vi "Write Error Handler Actor Queue.vi"(8 "error in (no error)":errorcluster, 10 "Actor Framework.lvlib:Message Enqueuer":refnum<class "Message Enqueuer.lvclass">, 11 "Controller in":refnum<class "Controller.lvclass">) -> (0 "error out":errorcluster, 3 "Controller out":refnum<class "Controller.lvclass">)   [LabVIEW 2026, in "Controller Actor.lvlib" / "Controller.lvclass"]
uses:
  Controller.lvclass
  Controller.lvclass/Controller.ctl
  <vilib>/ActorFramework/Message Enqueuer/Message Enqueuer.lvclass
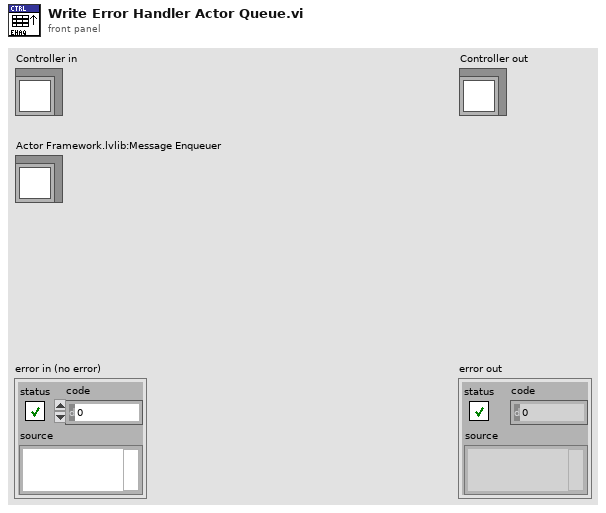
[diagram p1: front panel]
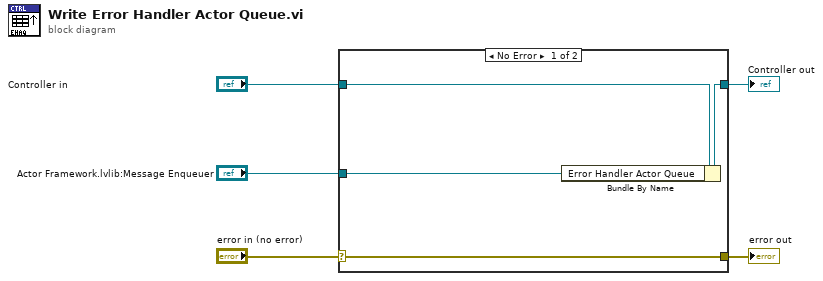
[diagram p0: block diagram]
diagram:
  n1 = case shown="No Error" "error in (no error)" {
    selector: "error in (no error)" -> [w9 w10]
    tunnel: [w9 w10] -> w4
    tunnel: [w7 w11] -> w2
    tunnel: "Controller in" -> [w8 w11]
    tunnel: "Actor Framework.lvlib:Message Enqueuer" -> [w6 _]
    frame No Error {
      n2 = Bundle By Name(cluster=w8, "Error Handler Actor Queue"=w6) -> (w7:refnum<class "Controller.lvclass">)
    }
    frame Error {
    }
  }
  "error out" <- w4
  "Controller out" <- w2
